vi "SortTimingPlotData.vi"(11 "TimingPlotData":T1[](array[typedef])) -> (3 "SortedTimingPlotData":T1[](array[typedef]))   [LabVIEW 2014]
uses:
  Controls/TimingPlotData.ctl
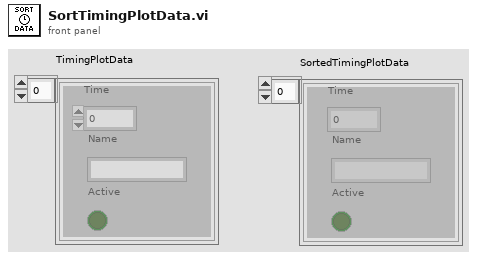
[diagram p1: front panel]
types:
  T1 = typedef "TimingPlotData.ctl" = cluster{"Time":dbl, "Name":string, "Active":bool}
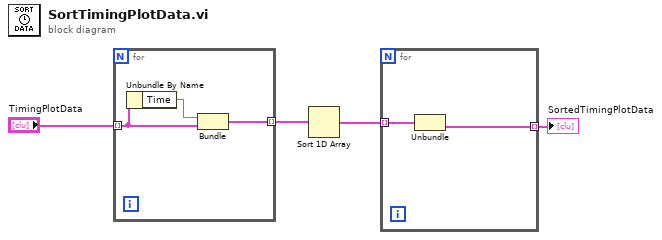
[diagram p0: block diagram]
diagram:
  n1 = for {
    tunnel: "TimingPlotData" -> [w6] mode=indexing
    tunnel: [w5] -> w3 mode=indexing
    n2 = Unbundle By Name(w6) -> ("Time"=w7:dbl)
    n3 = Bundle("Time"=w7, "TimingPlotData"=w6) -> (w5:cluster{"Time":dbl, "TimingPlotData":T1})  [unwired: 1 in]
  }
  n4 = Sort 1D Array(array=w3) -> (sorted array=w2:cluster{"Time":dbl, "TimingPlotData":T1}[])
  n5 = for {
    tunnel: w2 -> [w9] mode=indexing
    tunnel: [w8] -> w1 mode=indexing
    n6 = Unbundle(w9) -> ("TimingPlotData"=w8:T1)  [unwired: 1 out]
  }
  "SortedTimingPlotData" <- w1
